vi "Write Module Decimation.vi"(7 "Module ID":string, 8 "error in":errorcluster, 10 "Module Decimation":T1={"Decimation"=1, "Offset"=0, "sort order"=0, "async?"=FALSE}, 11 "Standard Engine Repo Data in":refnum<class "Standard Engine Configuration.lvclass">) -> (0 "error out":errorcluster, 3 "Standard Engine Repo Data out":refnum<class "Standard Engine Configuration.lvclass">)   [LabVIEW 2013, in "Standard Engine Configuration.lvclass"]
doc: "Specifies the decimation property of a specific module within the engine. A decimation value of 5 will inform the engine to call that module's methods every 5th execution cycle. The offset is a number ranging from 0-'Decimation' and specifies how many iterations pass before the engine calls that module's methods for the first time."
uses:
  Standard Engine Configuration.lvclass
  Module Decimation.ctl
  Standard Engine Configuration.lvclass/Standard Engine Configuration.ctl
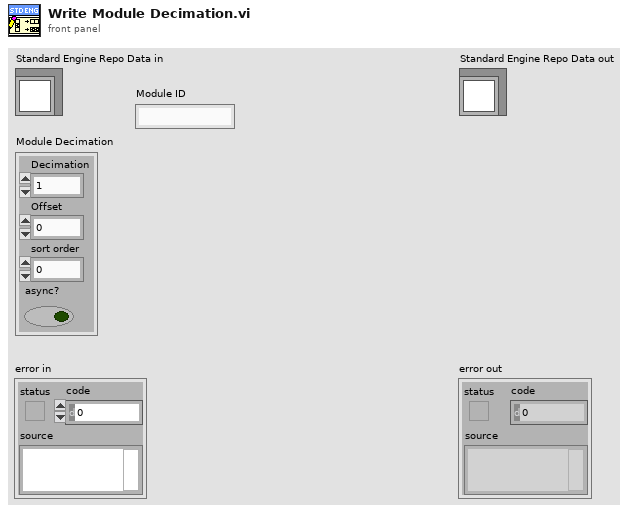
[diagram p1: front panel]
types:
  T1 = typedef "Standard Engine Configuration.lvclass/Module Decimation.ctl" = cluster{"Decimation":u16, "Offset":u16, "sort order":i32, "async?":bool}
  T2 = typedef "Standard Engine Configuration.lvclass/Module Specific Configuration.ctl" = cluster{"Module ID":string, "Module Decimation":T1, "error tag":string, "error responses":T3}
  T3 = typedef "Standard Engine Configuration.lvclass/error responses.ctl" = cluster{"unknown":T4, "trivial":T4, "critical":T4, "recoverable":T4}
  T4 = typedef "Standard Engine Configuration.lvclass/error options.ctl" = cluster{"clear":bool, "notify":bool, "remove module":bool, "abort engine":bool, "go to safe state":bool, "recover module":bool}
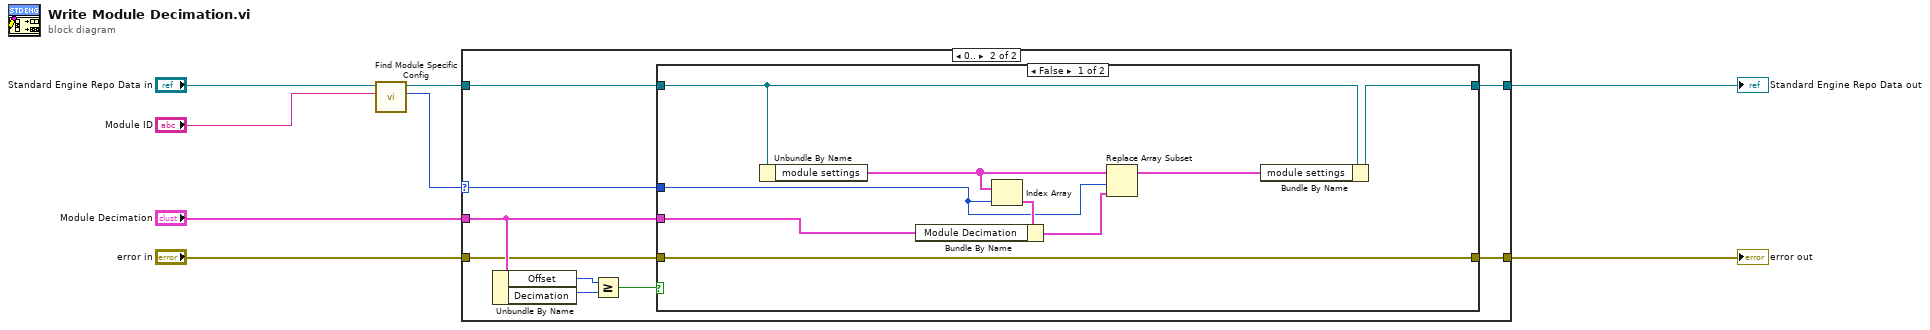
[diagram p0: block diagram]
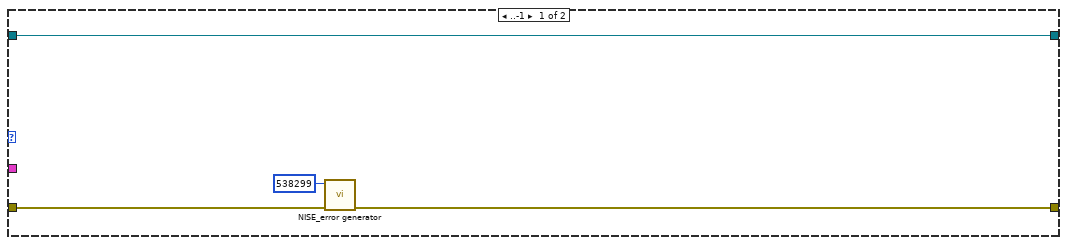
[diagram p2: hidden frame]
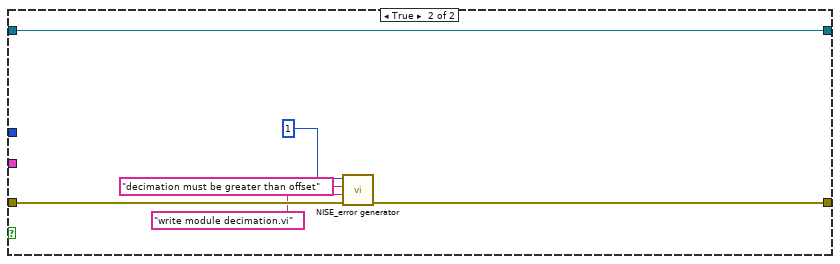
[diagram p3: hidden frame]
diagram:
  n1 = call "Find Module Specific Config.vi"("Module ID"="Module ID", "Standard Engine Repo Data in"="Standard Engine Repo Data in") -> ("Index"=w1:i32, "Standard Engine Repo Data out"=w2:refnum<class "Standard Engine Configuration.lvclass">)  [unwired: 8 in]
  n2 = case shown="0.." w1 {
    selector: w1 -> [_ w21]
    tunnel: w2 -> [w11 w20]
    tunnel: "error in" -> [w12 w13]
    tunnel: [w10 w14] -> w4
    tunnel: [w11 w19] -> w3
    tunnel: "Module Decimation" -> [_ w18]
    frame ..-1 {
      n3 = call <vilib>:"NISE_error generator.vi"("error in"=w12, "error code (0)"=538299) -> ("error out"=w10:errorcluster)  [unwired: 7 in]
    }
    frame 0.. {
      n4 = Unbundle By Name(w18) -> ("Offset"=w17:u16, "Decimation"=w16:u16)
      n5 = Greater Or Equal?(x=w17, y=w16) -> (x >= y?=w15:bool)
      n6 = case shown="False" w15 {
        tunnel: w21 -> [w29 _]
        tunnel: w20 -> [w26 w36]
        tunnel: [w24 w36] -> w19
        tunnel: w18 -> [w23 _]
        tunnel: [w22 w34] -> w14
        tunnel: w13 -> [w22 w35]
        frame False {
          n7 = Unbundle By Name(w26) -> ("module settings"=w28:T2[])
          n8 = Index Array(array=w28, index=w29) -> (element=w30:T2)
          n9 = Bundle By Name(cluster=w30, "Module Decimation"=w23) -> (w27:T2)
          n10 = Replace Array Subset(array=w28, new element=w27, index=w29) -> (w25:T2[])
          n11 = Bundle By Name(cluster=w26, "module settings"=w25) -> (w24:refnum<class "Standard Engine Configuration.lvclass">)
        }
        frame True {
          n12 = call <vilib>:"NISE_error generator.vi"("error in"=w35, "source"="write module decimation.vi", "append error message"="decimation must be greater than offset", "error code (0)"=1) -> ("error out"=w34:errorcluster)  [unwired: 5 in]
        }
      }
    }
  }
  "error out" <- w4
  "Standard Engine Repo Data out" <- w3
